vi "Finish.vi"(8 "error in (no error)":errorcluster, 11 "Receiver in":refnum<class "Receiver.lvclass">) -> (0 "error out":errorcluster, 3 "Receiver out":refnum<class "Receiver.lvclass">)   [LabVIEW 2013, in "Receiver.lvlib" / "Receiver.lvclass"]
uses:
  Receiver.lvclass
  System/System.lvclass
  Receiver.lvclass/Receiver.ctl
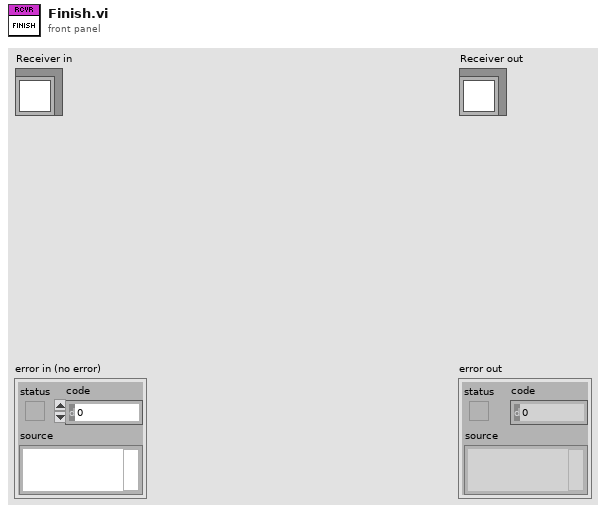
[diagram p1: front panel]
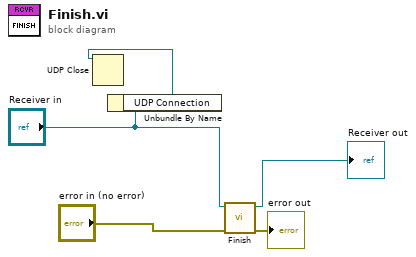
[diagram p0: block diagram]
diagram:
  n1 = Unbundle By Name("Receiver in") -> ("UDP Connection"=w2:refnum<k16>)
  n2 = UDP Close(connection ID=w2) -> ()  [unwired: 1 in, 2 out]
  n3 = call-parent "Finish.vi"("error in (no error)"="error in (no error)", "System in"="Receiver in") -> ("error out"=→"error out":errorcluster, "System out"=→"Receiver out":refnum<class "Receiver.lvclass">)  [unwired: 8 in]
